vi "Test Boards_TASK.vi"() -> ()   [LabVIEW 2018]
doc: "See <b>Read_Me.html</b> in the <b>Board Testing</b> project for a detailed description of this VI."
uses:
  Common/Board Image.ctl
  Classes/Assembly Line Input_class/Assembly Line Input.lvclass
panel:
  out "Test Results":T2(array[cluster])
  # "Overview: Demonstrates a task-based solution to a board testing problem.\n\nSee Read_Me.html in the project for a detailed description of this VI."
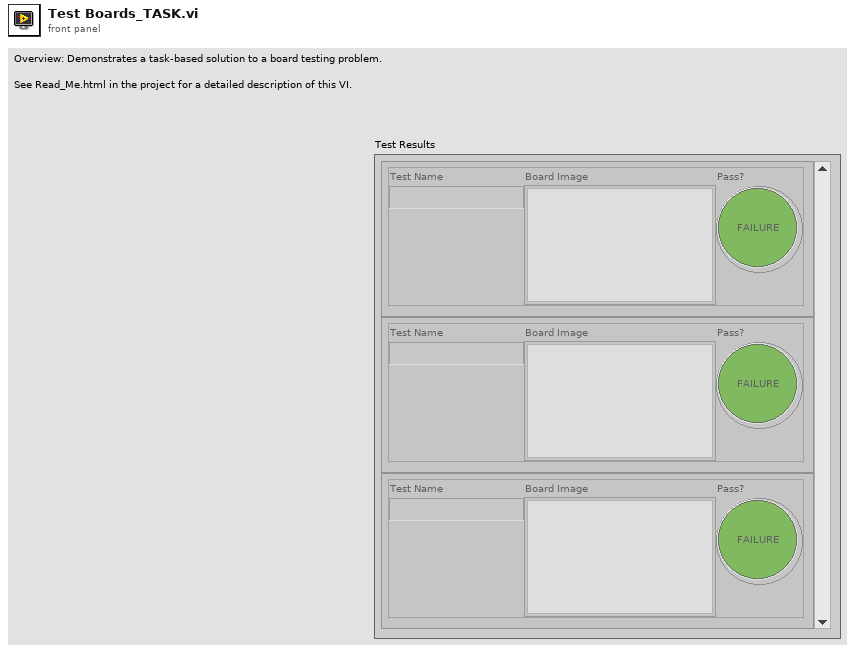
[diagram p1: front panel]
types:
  T1 = typedef "Board Image.ctl" = picture
  T2 = cluster{"Test Name":string, "Board Image":T1, "Pass?":bool}[]
  T3 = typedef "Board Type Enum.ctl" = enum16{"Basic DAQ Board", "Elite DAQ Board", "GPIB Board"}
  T4 = typedef "Pass Fail Boolean.ctl" = bool
  T5 = cluster{"test name":string, "Accessors:board image":T1, "Pass?":T4}
  T6 = cluster{"test name":string, "Accessors:board image":T1, "pass?":T4}
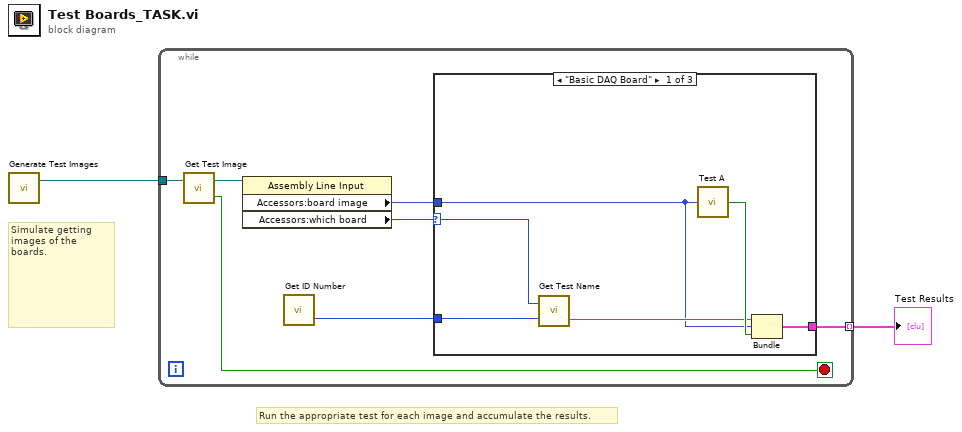
[diagram p0: block diagram]
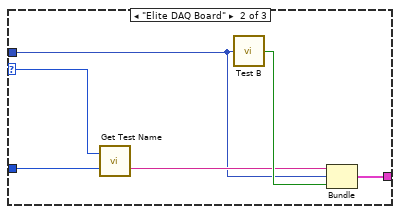
[diagram p2: hidden frame]
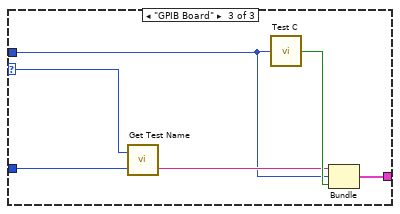
[diagram p3: hidden frame]
diagram:
  # "Run the appropriate test for each image and accumulate the results."
  # "Simulate getting images of the boards."
  n1 = call "Generate Test Images.vi"() -> ("queue out"=w2:refnum<queue>)  [unwired: 2 in, 1 out]
  n2 = while {
    tunnel: w2 -> [w9]
    tunnel: [w7] -> w1 mode=indexing
    stop <- w8 stop-if-true
    n3 = call "Get Test Image.vi"("queue in"=w9) -> ("no more images after this?"=w8:bool, "Assembly Line Input"=w5:refnum<class "Assembly Line Input.lvclass">)  [unwired: 1 in]
    n4 = property class="Assembly Line Input"(reference=w5) -> ("Accessors:board image"=w4:T1, "Accessors:which board"=w3:T3)  [unwired: 1 in, 2 out]
    n5 = call "Get ID Number.vi"() -> ("id number"=w6:u32)  [unwired: 2 in]
    n6 = case shown="\"Basic DAQ Board\"" w3 {
      selector: w3 -> [w15 w21 w27]
      tunnel: [w14 w20 w26] -> w7
      tunnel: w4 -> [w11 w17 w23]
      tunnel: w6 -> [w10 w16 w22]
      frame "Basic DAQ Board" {
        n7 = call "Get Test Name.vi"("id number"=w10, "which board"=w15) -> ("test name"=w12:string)  [unwired: 1 in]
        n8 = call "Test A.vi"("board image"=w11) -> ("Pass?"=w13:T4)
        n9 = Bundle("test name"=w12, "Accessors:board image"=w11, "Pass?"=w13) -> (w14:T5)  [unwired: 1 in]
      }
      frame "Elite DAQ Board" {
        n10 = call "Get Test Name.vi"("id number"=w16, "which board"=w21) -> ("test name"=w18:string)  [unwired: 1 in]
        n11 = call "Test B.vi"("board image"=w17) -> ("pass?"=w19:T4)
        n12 = Bundle("test name"=w18, "Accessors:board image"=w17, "pass?"=w19) -> (w20:T6)  [unwired: 1 in]
      }
      frame "GPIB Board" {
        n13 = call "Get Test Name.vi"("id number"=w22, "which board"=w27) -> ("test name"=w24:string)  [unwired: 1 in]
        n14 = call "Test C.vi"("board image"=w23) -> ("pass?"=w25:T4)
        n15 = Bundle("test name"=w24, "Accessors:board image"=w23, "pass?"=w25) -> (w26:T6)  [unwired: 1 in]
      }
    }
  }
  "Test Results" <- w1
